vi "4463 and 4464 sync test (4464 master).vi"() -> ()   [LabVIEW 2015]
uses:
  <vilib>/DAQmx/write.llb/DAQmx Write (Analog 1D DBL 1Chan NSamp).vi
  <vilib>/DAQmx/read.llb/DAQmx Read (Analog 1D DBL 1Chan NSamp).vi
  <vilib>/DAQmx/create/channels.llb/DAQmx Create Channel (AI-Voltage-Basic).vi
  <vilib>/DAQmx/configure/timing.llb/DAQmx Timing (Sample Clock).vi
  <vilib>/DAQmx/create/channels.llb/DAQmx Create Channel (AO-Voltage-Basic).vi
  <vilib>/DAQmx/configure/trigger.llb/DAQmx Start Trigger (Digital Edge).vi
  <vilib>/DAQmx/miscellaneous.llb/DAQmx Fill In Error Info.vi
  <resource>/objmgr/daqmx.rc
panel:
  out "Graph":dbl[](graph)
  in  "stop":bool
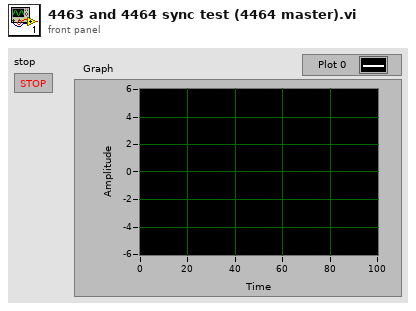
[diagram p1: front panel]
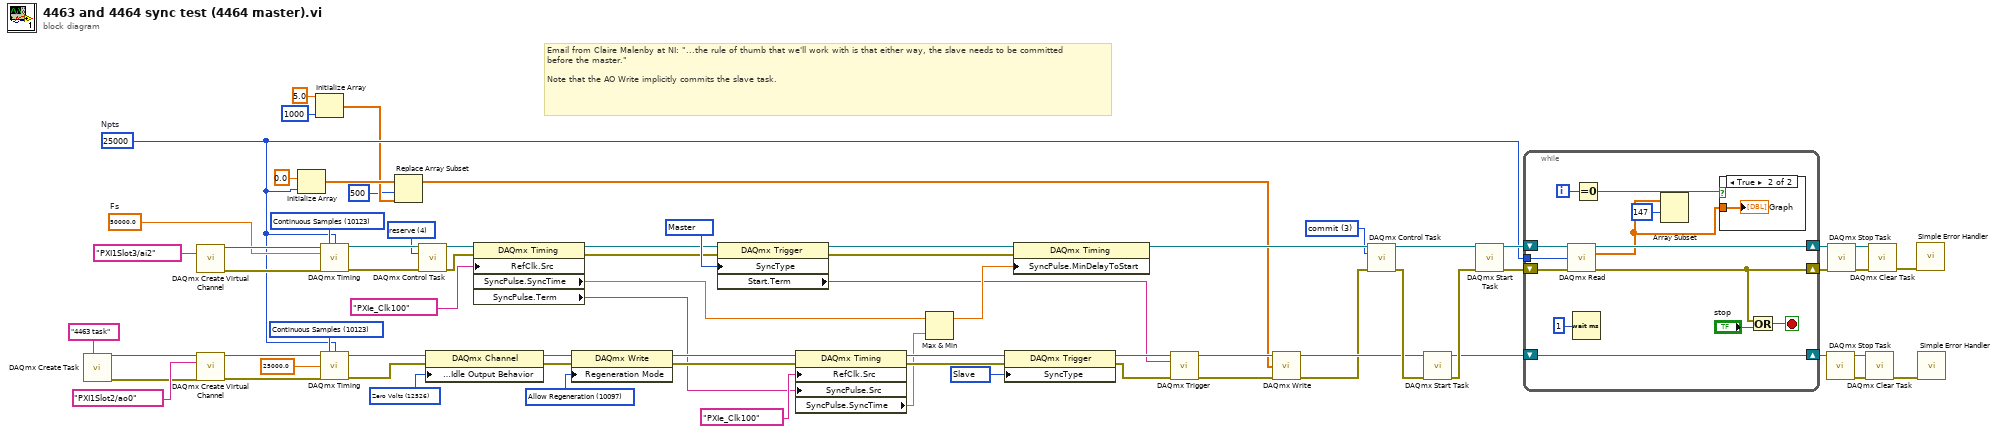
[diagram p0: block diagram]
diagram:
  w23 = 12526 items=["Zero Volts"=12526, "High-Impedance"=12527, "Maintain Existing Value"=12528] ("AO.IdleOutputBehavior")
  w26 = 3 items=["verify"=2, "reserve"=4, "commit"=3, "unreserve"=5, "abort"=6] ("action")
  w37 = 15888 items=["None"=10230, "Master"=15888, "Slave"=15889] ("SyncType")
  w38 = 15889 items=["None"=10230, "Master"=15888, "Slave"=15889] ("SyncType")
  w43 = 4 items=["verify"=2, "reserve"=4, "commit"=3, "unreserve"=5, "abort"=6] ("action")
  w14 = 50000.0  # Fs
  w66 = 10123 items=["Finite Samples"=10178, "Continuous Samples"=10123, "Hardware Timed Single Point"=12522] ("sample mode")
  w69 = 10097 items=["Allow Regeneration"=10097, "Do Not Allow Regeneration"=10158] ("RegenMode")
  w8 = 25000  # Npts
  w71 = 10123 items=["Finite Samples"=10178, "Continuous Samples"=10123, "Hardware Timed Single Point"=12522] ("sample mode")
  # "Email from Claire Malenby at NI: \"...the rule of thumb that we'll work with is that either way, the slave needs to be committed before the master.\"\n\nNote that the AO Write implicitly commits the slave task."
  n1 = call <vilib>:"DAQmx Create Task.vi"("new task name"="4463 task") -> ("task out"=w33:refnum<k21>, "error out"=w36:errorcluster)  [unwired: 13 in]
  n2 = call-poly <vilib>:"DAQmx Create Virtual Channel.vi"("physical channels"=tag "PXI1Slot3/ai2") -> ("task out"=w24:refnum<k21>, "error out"=w72:errorcluster)  [unwired: 13 in]
  n3 = call-poly <vilib>:"DAQmx Create Virtual Channel.vi"("task in"=w33, "physical channels"=tag "PXI1Slot2/ao0", "error in"=w36) -> ("task out"=w70:refnum<k21>, "error out"=w68:errorcluster)  [unwired: 11 in]
  n4 = Initialize Array(0.0 ("element"), w8) -> (w4:dbl[])
  n5 = Initialize Array(5.0 ("element"), 1000 ("element")) -> (w2:dbl[])
  n6 = call-poly <vilib>:"DAQmx Timing.vi"("task/channels in"=w24, "sample mode"=w71, "samples per channel"=w8, "rate"=w14, "error in"=w72) -> ("task out"=w47:refnum<k21>, "error out"=w46:errorcluster)  [unwired: 9 in]
  n7 = call-poly <vilib>:"DAQmx Timing.vi"("task/channels in"=w70, "sample mode"=w66, "samples per channel"=w8, "rate"=25000.0, "error in"=w68) -> ("task out"=w18:refnum<k21>, "error out"=w16:errorcluster)  [unwired: 9 in]
  n8 = Replace Array Subset(array=w4, new element=w2, index=500) -> (w3:dbl[])
  n9 = call <vilib>:"DAQmx Control Task.vi"("task/channels in"=w47, "action"=w43, "error in"=w46) -> ("task out"=w44:refnum<k21>, "error out"=w45:errorcluster)  [unwired: 11 in]
  n10 = property class="DAQmx Channel"(reference=w18, error in=w16, "Analog Output:General Properties:Output Configuration:Idle Output Behavior"=w23) -> (reference out=w17:refnum<k21>, error out=w15:errorcluster)
  n11 = property class="DAQmx Timing"(reference=w44, error in=w45, "RefClk.Src"=tag "PXIe_Clk100") -> (reference out=w21:refnum<k21>, error out=w30:errorcluster, "SyncPulse.SyncTime"=w13:dbl, "SyncPulse.Term"=w34:tag)
  n12 = property class="DAQmx Write"(reference=w17, error in=w15, "Regeneration Mode"=w69) -> (reference out=w65:refnum<k21>, error out=w64:errorcluster)
  n13 = property class="DAQmx Trigger"(reference=w21, error in=w30, "SyncType"=w37) -> (reference out=w9:refnum<k21>, error out=w12:errorcluster, "Start.Term"=w11:tag)
  n14 = property class="DAQmx Timing"(reference=w65, error in=w64, "RefClk.Src"=tag "PXIe_Clk100", "SyncPulse.Src"=w34) -> (reference out=w42:refnum<k21>, error out=w41:errorcluster, "SyncPulse.SyncTime"=w29:dbl)
  n15 = Max & Min(x=w13, y=w29) -> (max(x,y)=w28:dbl)  [unwired: 1 out]
  n16 = property class="DAQmx Trigger"(reference=w42, error in=w41, "SyncType"=w38) -> (reference out=w40:refnum<k21>, error out=w39:errorcluster)
  n17 = property class="DAQmx Timing"(reference=w9, error in=w12, "SyncPulse.MinDelayToStart"=w28) -> (reference out=w27:refnum<k21>)  [unwired: 1 out]
  n18 = call-poly <vilib>:"DAQmx Trigger.vi"("task/channels in"=w40, "source"=w11, "error in"=w39) -> ("task out"=w51:refnum<k21>, "error out"=w52:errorcluster)  [unwired: 11 in]
  n19 = call-poly <vilib>:"DAQmx Write.vi"("task/channels in"=w51, "data"=w3, "error in"=w52) -> ("task out"=w20:refnum<k21>, "error out"=w19:errorcluster)  [unwired: 10 in, 1 out]
  n20 = call <vilib>:"DAQmx Control Task.vi"("task/channels in"=w27, "action"=w26, "error in"=w19) -> ("task out"=w32:refnum<k21>, "error out"=w31:errorcluster)  [unwired: 11 in]
  n21 = call <vilib>:"DAQmx Start Task.vi"("task/channels in"=w20, "error in"=w31) -> ("task out"=w60:refnum<k21>, "error out"=w63:errorcluster)  [unwired: 12 in]
  n22 = call <vilib>:"DAQmx Start Task.vi"("task/channels in"=w32, "error in"=w63) -> ("task out"=w61:refnum<k21>, "error out"=w62:errorcluster)  [unwired: 12 in]
  n23 = while {
    tunnel: w8 -> [w79]
    shift-right: [w77] -> w58
    shift-left: w62 -> [w81]
    shift-right: [w83] -> w57
    shift-left: w60 -> [w83]
    shift-right: [w80] -> w59
    shift-left: w61 -> [w82]
    i -> [w76]
    stop <- w78 stop-if-true
    n24 = call-poly <vilib>:"DAQmx Read.vi"("task/channels in"=w82, "number of samples per channel"=w79, "error in"=w81) -> ("task out"=w80:refnum<k21>, "data"=w73:dbl[], "error out"=w77:errorcluster)  [unwired: 10 in]
    n25 = Wait (ms)(milliseconds to wait=u32 1) -> ()  [unwired: 1 out]
    n26 = Equal To 0?(x=w76) -> (x = 0?=w75:bool)
    n27 = Array Subset(array=w73, index=147) -> ()  [unwired: 1 in, 1 out]
    n28 = case shown="True" w75 {
      tunnel: w73 -> [_ w86]
      frame False {
      }
      frame True {
        "Graph" <- w86
      }
    }
    n29 = Or(x=w77, y="stop") -> (x .or. y?=w78:bool)
  }
  n30 = call <vilib>:"DAQmx Stop Task.vi"("task/channels in"=w57) -> ("task out"=w54:refnum<k21>, "error out"=w53:errorcluster)  [unwired: 13 in]
  n31 = call <vilib>:"DAQmx Stop Task.vi"("task/channels in"=w59, "error in"=w58) -> ("task out"=w56:refnum<k21>, "error out"=w55:errorcluster)  [unwired: 12 in]
  n32 = call <vilib>:"DAQmx Clear Task.vi"("task in"=w54, "error in"=w53) -> ("error out"=w48:errorcluster)  [unwired: 13 in]
  n33 = call <vilib>:"DAQmx Clear Task.vi"("task in"=w56, "error in"=w55) -> ("error out"=w22:errorcluster)  [unwired: 13 in]
  n34 = call <vilib>:"Simple Error Handler.vi"("error in (no error)"=w22) -> ()  [unwired: 4 in, 5 out]
  n35 = call <vilib>:"Simple Error Handler.vi"("error in (no error)"=w48) -> ()  [unwired: 4 in, 5 out]
